vi "Read Done.vi"(8 "error in (no error)":errorcluster, 11 "CorrFactor in":refnum<class "CorrFactor.lvclass">) -> (0 "error out":errorcluster, 2 "Done":bool, 3 "CorrFactor out":refnum<class "CorrFactor.lvclass">)   [LabVIEW 2018, in "AnalysisPlugins.lvlib" / "CorrFactor.lvclass"]
uses:
  CorrFactor.lvclass
  CorrFactor.lvclass/CorrFactor.ctl
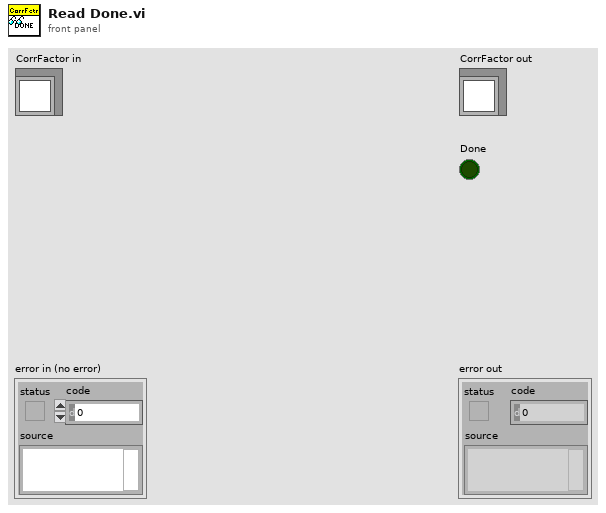
[diagram p1: front panel]
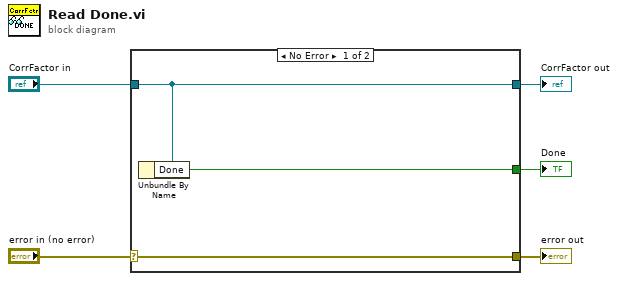
[diagram p0: block diagram]
diagram:
  n1 = case shown="No Error" "error in (no error)" {
    selector: "error in (no error)" -> [w8 w9]
    tunnel: [w8 w9] -> w4
    tunnel: [w7 w10] -> w2
    tunnel: "CorrFactor in" -> [w7 w10]
    tunnel: [w6 _] -> w1
    frame No Error {
      n2 = Unbundle By Name(w7) -> ("Done"=w6:bool)
    }
    frame Error {
    }
  }
  "error out" <- w4
  "CorrFactor out" <- w2
  "Done" <- w1
